vi "Pre Launch Init.vi"(11 "Caller in":refnum<class "Nested.lvclass">) -> (0 "error out":errorcluster, 3 "Caller out":refnum<class "Nested.lvclass">)   [LabVIEW 2020, in "Nested.lvlib" / "Nested.lvclass"]
doc: "(<B>Filename</B>: Actor Framework.lvlib:Actor.lvclass:Pre Launch Init.vi)\n\nDefines behavior that occurs after the Launch Nested Actor method is invoked but before the actor's Actor Core method begins running.\n\nBy default, this method does nothing. A descendant class may override it to define behavior."
uses:
  Nested.lvclass
  C:/Program Files/National Instruments/LabVIEW 2020/vi.lib/ActorFramework/Actor/Actor.lvclass
  Nested.lvclass/Nested.ctl
  <vilib>/ActorFramework/Actor/Actor.lvclass/Actor.ctl
  <vilib>/ActorFramework/Message Enqueuer/Message Enqueuer.lvclass/Message Enqueuer.ctl
  <vilib>/ActorFramework/Message Enqueuer/Init from Existing Queue.vi
  <vilib>/ActorFramework/Actor/Actor.lvclass
  <vilib>/ActorFramework/Message Enqueuer/Message Enqueuer.lvclass
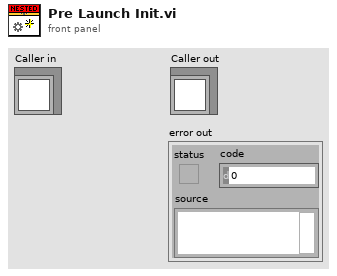
[diagram p1: front panel]
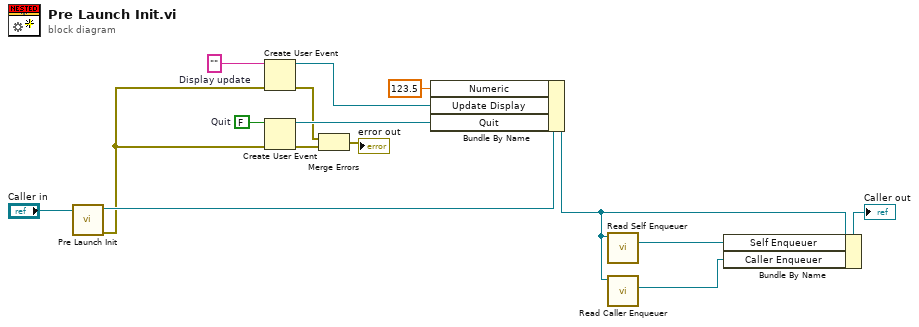
[diagram p0: block diagram]
diagram:
  w8 = ""  # Display update
  w15 = FALSE  # Quit
  n1 = call-parent "Pre Launch Init.vi"("Actor in"="Caller in") -> ("error out"=w7:errorcluster, "Actor out"=w10:refnum<class "Nested.lvclass">)  [unwired: 9 in]
  n2 = Create User Event(user event datatype=w8, error in=w7) -> (user event=w4:refnum<user-event>, error out=w5:errorcluster)
  n3 = Create User Event(user event datatype=w15, error in=w7) -> (user event=w14:refnum<user-event>, error out=w9:errorcluster)
  n4 = Merge Errors(w5, w9) -> (→"error out":errorcluster)
  n5 = Bundle By Name(cluster=w10, "Numeric"=123.5, "Update Display"=w4, "Quit"=w14) -> (w2:refnum<class "Nested.lvclass">)
  n6 = call <vilib>:"Read Self Enqueuer.vi"("Actor"=w2) -> ("Self Enqueuer"=w12:refnum<class "Message Enqueuer.lvclass">)  [unwired: 10 in]
  n7 = call <vilib>:"Read Caller Enqueuer.vi"("Actor"=w2) -> ("Caller Enqueuer"=w1:refnum<class "Message Enqueuer.lvclass">)  [unwired: 10 in]
  n8 = Bundle By Name(cluster=w2, "Self Enqueuer"=w12, "Caller Enqueuer"=w1) -> (→"Caller out":refnum<class "Nested.lvclass">)
